vi "Update_DB_for_new_file_loc.vi"() -> ()   [LabVIEW 2013]
uses:
  Controls/File_location.ctl
  <vilib>/addons/database/Connection.llb/Conn Execute.vi
  <vilib>/addons/database/Recordset.llb/Rec Destroy - Connection.vi
  <vilib>/addons/database/NI_Database_API.lvlib
panel:
  in  "error in (no error)":errorcluster
  out "error out":errorcluster
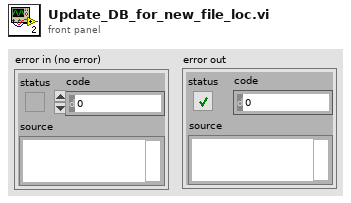
[diagram p1: front panel]
types:
  T1 = typedef "File_location.ctl" = i8
  T2 = typedef "NI_Database_API.lvlib/Conn ObjectReference.ctl" = refnum<k1>
  T3 = typedef "NI_Database_API.lvlib/Rec ObjectReference.ctl" = refnum<k1>
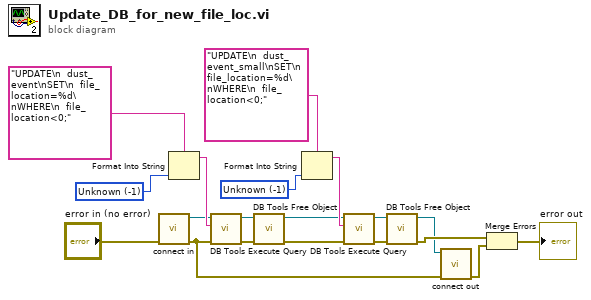
[diagram p0: block diagram]
diagram:
  w5 = T1 -1 items=["Unknown"=-1, "Processing"=0, "Storage"=1] ("File Location")
  w19 = T1 -1 items=["Unknown"=-1, "Processing"=0, "Storage"=1] ("File Location")
  n1 = call "connect in.vi"("error in (no error)"="error in (no error)") -> ("error out"=w14:errorcluster, "Database Connection"=w15:T2)  [unwired: 6 in, 1 out]
  n2 = Format Into String(format string="UPDATE\n  dust_event\nSET\n  file_location=%d\nWHERE\n  file_location<0;", w19) -> (resulting string=w18:string)  [unwired: 2 in, 1 out]
  n3 = call-poly <vilib>:"DB Tools Execute Query.vi"("error in (no error)"=w14, "SQL query"=w18, "connection reference"=w15) -> ("error out"=w16:errorcluster, "recordset reference"=w17:T3)  [unwired: 5 in]
  n4 = call-poly <vilib>:"DB Tools Free Object.vi"("error in (no error)"=w16, "recordset reference"=w17) -> ("error out"=w4:errorcluster, "connection reference"=w1:T2)  [unwired: 8 in]
  n5 = Format Into String(format string="UPDATE\n  dust_event_small\nSET\n  file_location=%d\nWHERE\n  file_location<0;", w5) -> (resulting string=w6:string)  [unwired: 2 in, 1 out]
  n6 = call-poly <vilib>:"DB Tools Execute Query.vi"("error in (no error)"=w4, "SQL query"=w6, "connection reference"=w1) -> ("error out"=w8:errorcluster, "recordset reference"=w7:T3)  [unwired: 5 in]
  n7 = call-poly <vilib>:"DB Tools Free Object.vi"("error in (no error)"=w8, "recordset reference"=w7) -> ("error out"=w3:errorcluster, "connection reference"=w2:T2)  [unwired: 8 in]
  n8 = call "connect out.vi"("error in (no error)"=w14, "connection reference"=w2) -> ("error out"=w13:errorcluster)  [unwired: 9 in]
  n9 = Merge Errors(w3, w13) -> (→"error out":errorcluster)
